vi "filterwheelcontrol.vi"(11 "ODfilt":u16(ring)=1 caption="IR laser OD value" items=["OD 0"=1, "OD 0.5"=2, "OD 1"=3, "OD 2"=4, "OD 3"=5, "OD 4"=6]) -> ()   [LabVIEW 2015]
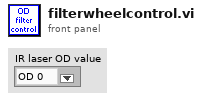
[diagram p1: front panel]
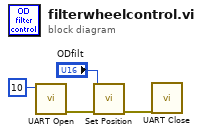
[diagram p0: block diagram]
diagram:
  n1 = call "UART Open.vi"("Serial Port"=10) -> ("error out"=w4:errorcluster)  [unwired: 9 in, 1 out]
  n2 = call "Set Position.vi"("error in (no error)"=w4, "Position"="ODfilt") -> ("error out"=w3:errorcluster)  [unwired: 9 in]
  n3 = call "UART Close.vi"("error in (no error)"=w3) -> ()  [unwired: 10 in, 1 out]
